vi "Post Media Tweet - From LabVIEW Picture Type.vi"(8 "error in":errorcluster, 9 "LabVIEW Picture Type":picture, 10 "Tweet":string, 11 "Twitter Handle In":T1={"OAuth Credentials"={"Consumer Key"="", "Signature Method"=enum."HMAC-SHA1", "Token"="", "Version"="", "Token Secret"="", "Consumer Secret"=""}, "since ID"="", "max ID"="", "Screen Name"=""}) -> (0 "error out":errorcluster, 3 "Twitter Handle Out":T1={"OAuth Credentials"={"Consumer Key"="", "Signature Method"=enum."HMAC-SHA1", "Token"="", "Version"="", "Token Secret"="", "Consumer Secret"=""}, "since ID"="", "max ID"="", "Screen Name"=""})   [LabVIEW 2011, in "i3-twitter.lvlib"]
uses:
  i3-twitter.lvlib
  Controls/Twitter Handle.ctl
  i3-oauth/Controls/OAuth Credentials.ctl
  i3-oauth/Controls/Signature Method.ctl
  <vilib>/httpClient/MultipartData.ctl
  i3-oauth/Controls/HTTP Method.ctl
  i3-oauth/i3-oauth.lvlib
  <vilib>/httpClient/LabVIEWHTTPClient.lvlib
  <vilib>/wsapi/NI_WebServices.lvlib
panel:
  out "headers (response)":string
  out "body (response)":string
  out "Header Value":string
  out "Full URL":string
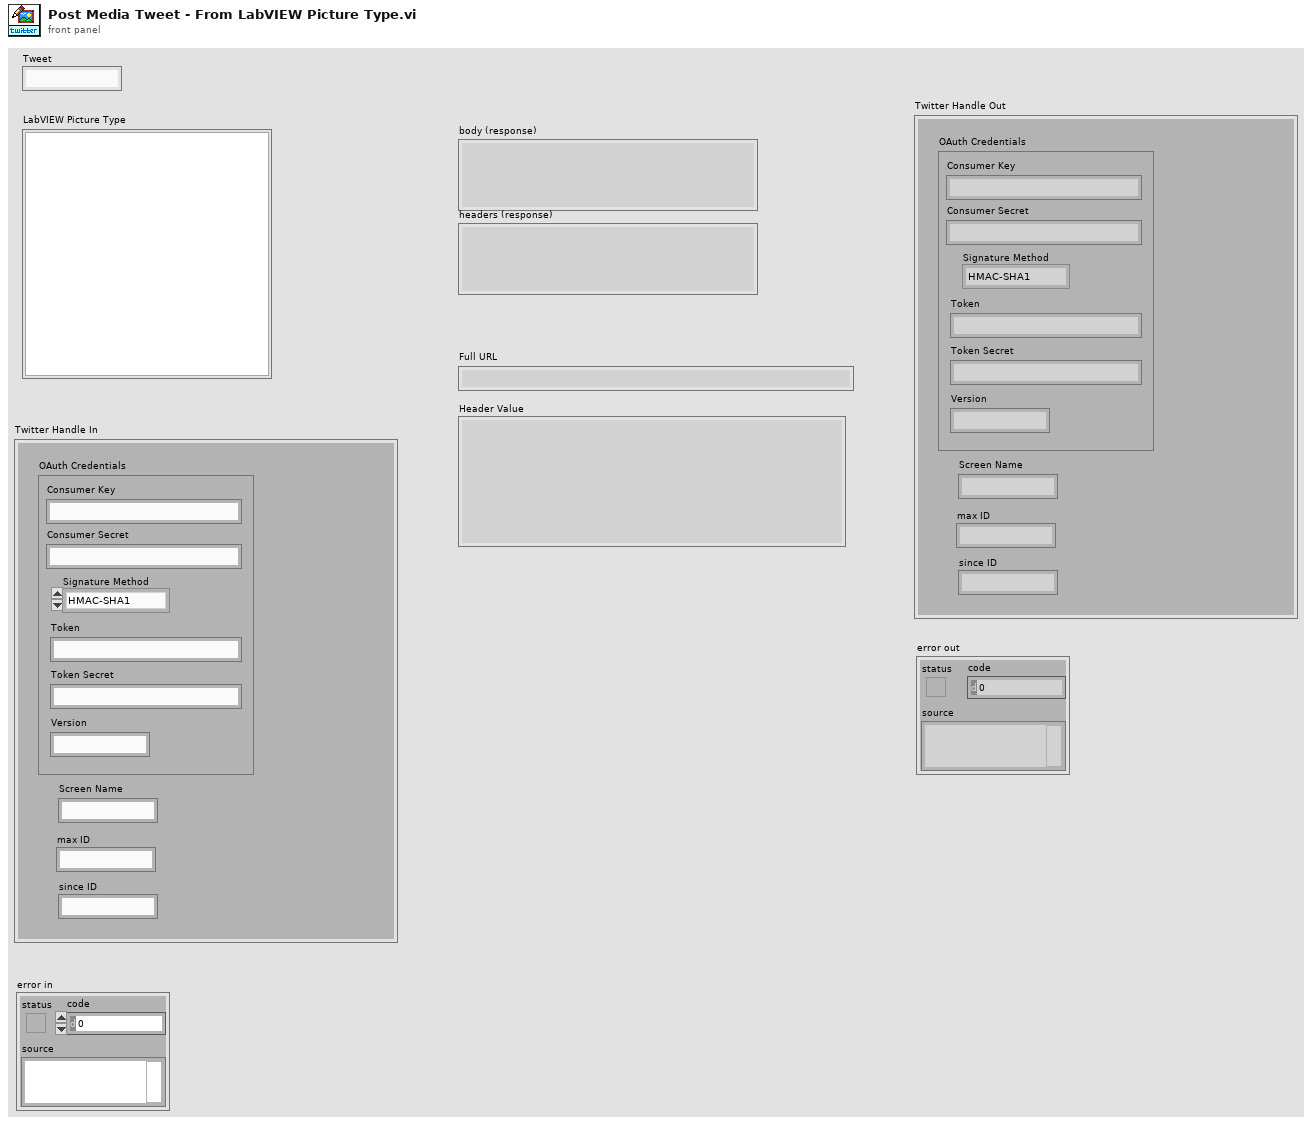
[diagram p1: front panel]
types:
  T1 = typedef "i3-twitter.lvlib/Twitter Handle.ctl" = cluster{"OAuth Credentials":T2, "since ID":string, "max ID":string, "Screen Name":string}
  T2 = typedef "i3-oauth.lvlib/OAuth Credentials.ctl" = cluster{"Consumer Key":string, "Signature Method":T3, "Token":string, "Version":string, "Token Secret":string, "Consumer Secret":string}
  T3 = typedef "i3-oauth.lvlib/Signature Method.ctl" = enum16{"HMAC-MD5", "HMAC-SHA1", "HMAC-SHA224", "HMAC-SHA256", "HMAC-SHA384", "HMAC-SHA512"}
  T4 = typedef "LabVIEWHTTPClient.lvlib/MultipartData.ctl" = cluster{"Name":string, "Value":string, "File":path, "Filename":string, "MIME type":string}
  T5 = typedef "i3-oauth.lvlib/HTTP Method.ctl" = enum16{"GET", "POST", "PUT", "DELETE"}
  T6 = typedef "imagedata.ctl" = cluster{"image type":i32, "image depth":i32, "image":u8[], "mask":u8[], "colors":u32[], "Rectangle":cluster{"left":i16, "top":i16, "right":i16, "bottom":i16}}
  T7 = cluster{"left":i16, "top":i16, "right":i16, "bottom":i16}
  T8 = typedef "LabVIEWHTTPClient.lvlib/ClientHandle.ctl" = refnum<k1>
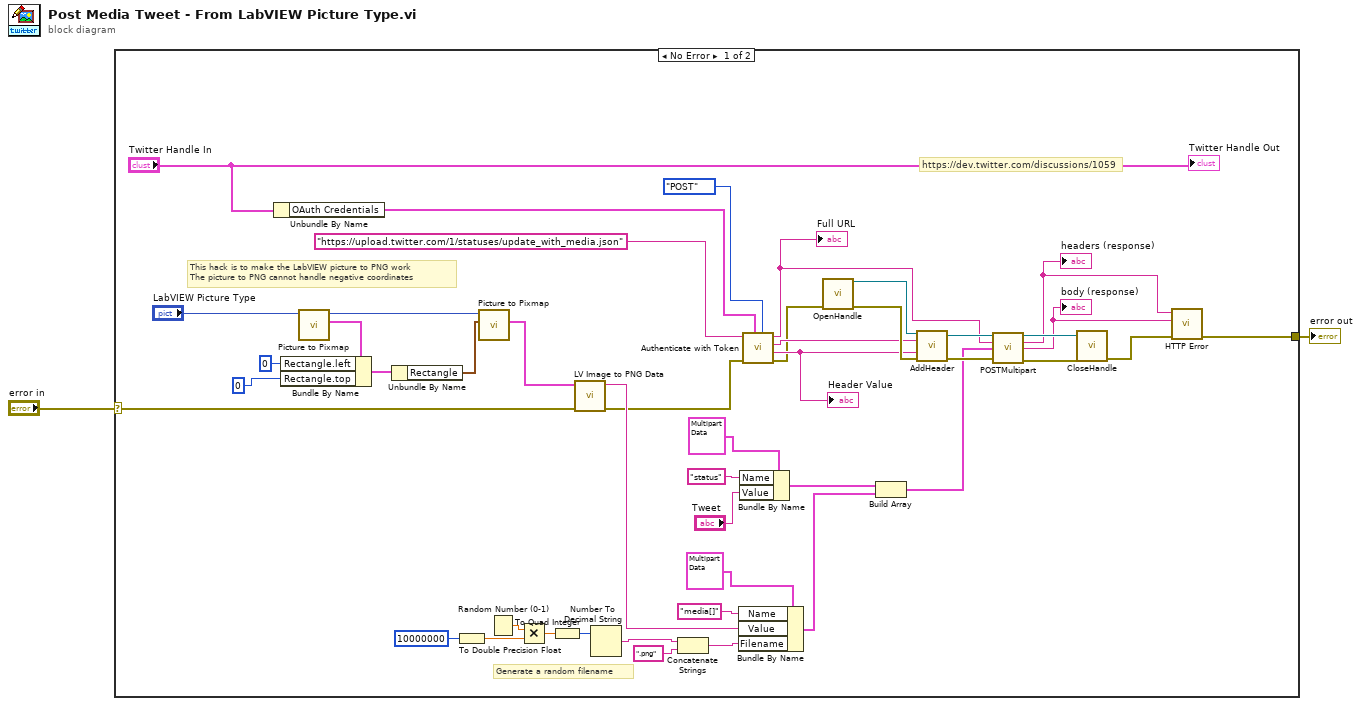
[diagram p0: block diagram]
diagram:
  n1 = case shown="No Error" "error in" {
    selector: "error in" -> [w4 w48]
    tunnel: [w5 w48] -> w2
    frame No Error {
      # "Generate a random filename"
      # "This hack is to make the LabVIEW picture to PNG work\nThe picture to PNG cannot handle negative coordinates"
      # "https://dev.twitter.com/discussions/1059"
      n2 = Unbundle By Name("Twitter Handle In") -> ("OAuth Credentials"=w15:T2)
      n3 = call <vilib>:"Picture to Pixmap.vi"("picture"="LabVIEW Picture Type") -> ("image data"=w23:T6, "new picture"=w27:picture)  [unwired: 9 in]
      n4 = Bundle By Name(cluster=w23, "Rectangle.left"=i16 0, "Rectangle.top"=i16 0) -> (w26:T6)
      n5 = Unbundle By Name(w26) -> ("Rectangle"=w28:T7)
      n6 = To Double Precision Float(number=10000000) -> (double precision float=w18:dbl)
      n7 = call <vilib>:"Picture to Pixmap.vi"("rect"=w28, "picture"=w27) -> ("image data"=w29:T6)  [unwired: 8 in, 1 out]
      n8 = Random Number (0-1)() -> (number: 0 to 1=w20:dbl)
      n9 = Multiply(x=w20, y=w18) -> (x*y=w8:dbl)
      n10 = To Quad Integer(1:w8) -> (0:w7:i64)
      n11 = call <vilib>:"LV Image to PNG Data.vi"("error in (no error)"=w4, "image data"=w29) -> ("error out"=w21:errorcluster, "png data"=w22:string)  [unwired: 8 in]
      n12 = Number To Decimal String(number=w7) -> (decimal integer string=w11:string)  [unwired: 1 in]
      n13 = Concatenate Strings(w11, ".png" ("string")) -> (w9:string)
      n14 = Bundle By Name(cluster=T4 {"Name"="", "Value"="", "File"=path "", "Filename"="", "MIME type"="application/octet-stream"} ("Element"), "Name"="media[]", "Value"=w22, "Filename"=w9) -> (w32:T4)
      n15 = Bundle By Name(cluster=T4 {"Name"="", "Value"="", "File"=path "", "Filename"="", "MIME type"="application/octet-stream"} ("Element"), "Name"="status", "Value"="Tweet") -> (w36:T4)
      n16 = call "Authenticate with Token.vi"("HTTP Method"=HTTP_Method."POST", "OAuth Credentials"=w15, "error in (no error)"=w21, "Base URL"="https://upload.twitter.com/1/statuses/update_with_media.json") -> ("error out"=w6:errorcluster, "Header Value"=w43:string, "Header Parameter"=w44:string, "Full URL"=w38:string)  [unwired: 3 in, 1 out]
      "Full URL" <- w38
      "Header Value" <- w43
      n17 = call <vilib>:"OpenHandle.vi"("error in (no error)"=w6) -> ("client handle out"=w46:T8, "error out"=w45:errorcluster)  [unwired: 13 in]
      n18 = Build Array(w36, w32) -> (w35:T4[])
      n19 = call <vilib>:"AddHeader.vi"("client handle"=w46, "header"=w44, "value"=w43, "error in (no error)"=w45) -> ("client handle out"=w42:T8, "error out"=w41:errorcluster)  [unwired: 10 in]
      n20 = call <vilib>:"POSTMultipart.vi"("client handle"=w42, "url"=w38, "data"=w35, "error in (no error)"=w41) -> ("client handle out"=w39:T8, "headers"=w12:string, "body"=w13:string, "error out"=w40:errorcluster)  [unwired: 8 in]
      "body (response)" <- w13
      "headers (response)" <- w12
      n21 = call <vilib>:"CloseHandle.vi"("client handle"=w39, "error in (no error)"=w40) -> ("error out"=w14:errorcluster)  [unwired: 13 in]
      n22 = call "HTTP Error.vi"("error in (no error)"=w14, "Body"=w13, "Header"=w12) -> ("error out"=w5:errorcluster)  [unwired: 6 in, 2 out]
      "Twitter Handle Out" <- "Twitter Handle In"
    }
    frame Error {
    }
  }
  "error out" <- w2
